vi "Command ADC.vi"(0 "Serial Devices in":refnum<class "Serial Devices.lvclass">, 1 "Device":string, 7 "Chanel":u8, 11 "error in (no error)":errorcluster) -> (4 "Serial Devices out":refnum<class "Serial Devices.lvclass">, 6 "Command":string, 10 "Expected":string, 15 "error out":errorcluster)   [LabVIEW 2019, in "Serial Devices.lvlib" / "Serial Devices.lvclass"]
uses:
  Serial Devices.lvclass
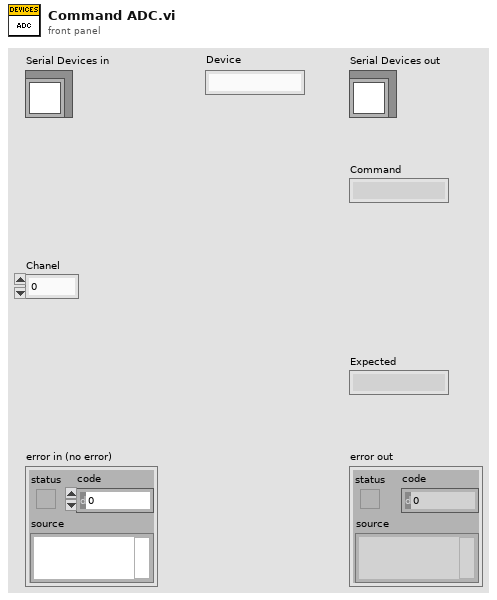
[diagram p1: front panel]
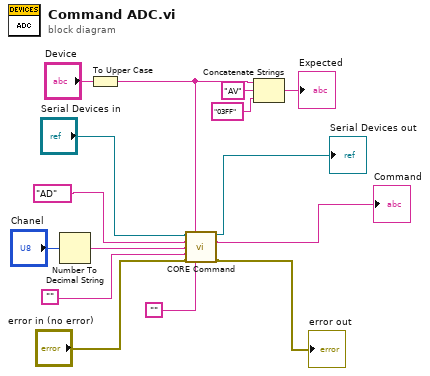
[diagram p0: block diagram]
diagram:
  n1 = Number To Decimal String(number="Chanel") -> (decimal integer string=w7:string)  [unwired: 1 in]
  n2 = To Upper Case(1:"Device") -> (0:w3:string)
  n3 = call "CORE Command.vi"("Serial Devices in"="Serial Devices in", "Device"=w3, "Command"="AD", "Chanel-Puerto"=w7, "Param-Pin"="", "error in (no error)"="error in (no error)", "Valor"="") -> ("Serial Devices out"=→"Serial Devices out":refnum<class "Serial Devices.lvclass">, "Command"=→"Command":string, "error out"=→"error out":errorcluster)  [unwired: 5 in, 1 out]
  n4 = Concatenate Strings(w3, "AV" ("string"), "03FF" ("string")) -> (→"Expected":string)
